vi "p1.vi"() -> ()   [LabVIEW 2015]
panel:
  in  "login":bool
  in  "Stop Button":bool
  in  "Color Box 2":u32(colorbox)
  in  "Boolean 2":bool
  out "Waveform Graph 2":i32[](graph)
  in  "Password":string
  in  "User Name":string
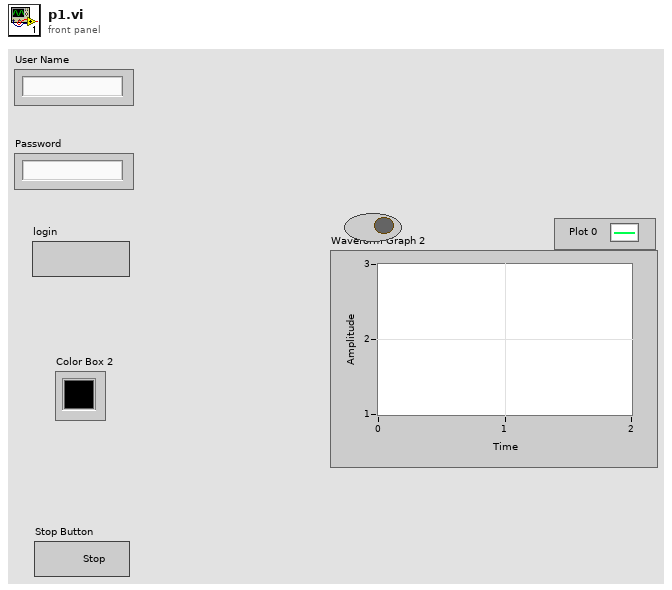
[diagram p1: front panel]
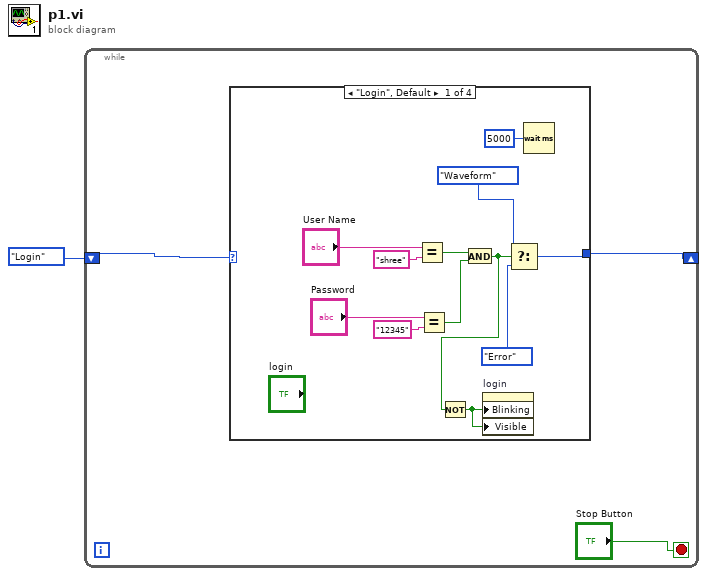
[diagram p0: block diagram]
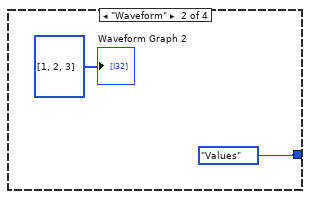
[diagram p2: hidden frame]
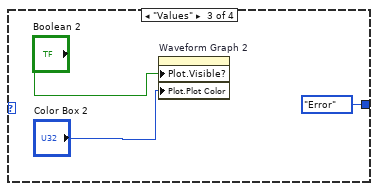
[diagram p3: hidden frame]
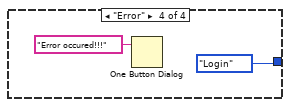
[diagram p4: hidden frame]
diagram:
  n1 = while {
    shift-right: [w4] -> _
    shift-left: enum16{"Login", "Waveform", "Values", "Error"}."Login" -> [w3]
    stop <- "Stop Button" stop-if-true
    n2 = case shown="\"Login\", Default" w3 {
      tunnel: [w10 enum16{"Login", "Waveform", "Values", "Error"}."Values" enum16{"Login", "Waveform", "Values", "Error"}."Error" enum16{"Login", "Waveform", "Values", "Error"}."Login"] -> w4
      frame "Login", Default {
        n3 = Equal?(x="User Name", y="shree" ("regular expression")) -> (x = y?=w11:bool)
        n4 = Equal?(x="Password", y="12345") -> (x = y?=w12:bool)
        n5 = And(x=w11, y=w12) -> (x .and. y?=w5:bool)
        n6 = Not(x=w5) -> (.not. x?=w6:bool)
        n7 = property on="login" class="Bool"("Blinking"=w6, "Visible"=w6) -> ()  [unwired: 2 in, 2 out]
        n8 = Select(t=enum16{"Login", "Waveform", "Values", "Error"}."Waveform", s=w5, f=enum16{"Login", "Waveform", "Values", "Error"}."Error") -> (s? t:f=w10:enum16{"Login", "Waveform", "Values", "Error"})
        n9 = Wait (ms)(milliseconds to wait=u32 5000) -> ()  [unwired: 1 out]
      }
      frame "Waveform" {
        "Waveform Graph 2" <- i32[] [1, 2, 3]
      }
      frame "Values" {
        n10 = property on="Waveform Graph 2" class="WFGraph (strict)"("Plot.Visible?"="Boolean 2", "Plot.Plot Color"="Color Box 2") -> ()  [unwired: 2 in, 2 out]
      }
      frame "Error" {
        n11 = One Button Dialog(message="Error occured!!!") -> ()  [unwired: 1 in, 1 out]
      }
    }
  }
